vi "BodeMagnitudePlot.vi"() -> ()   [LabVIEW 2014]
uses:
  <vilib>/imath/engines/lvmath2/RunTimeEngine/Managers/WorkSpace/UID Generator.vi
  <vilib>/imath/engines/lvmath2/RunTimeEngine/RunTimeType/NIMS_RunTimeType_From StrictType (excl LVString).vi
  <instcachedir>/0/NIMS_RunTimeType_From StrictType (excl LVString)_15A5391EEA9C4AACB9955AC755B83D29.lvgen/NIMS_RunTimeType_From StrictType (excl LVString)_15A5391EEA9C4AACB9955AC755B83D29_000.vi
  <vilib>/imath/engines/lvmath2/RunTimeEngine/LocalVariableDefStatement/MC_LocalVariableDefStatement_Display.vi
  <vilib>/imath/engines/lvmath2/RunTimeEngine/Managers/SymbolTable/Clear UID.vi
  <vilib>/imath/engines/lvmath2/RunTimeEngine/NodeEndStatement/NIMS_NodeEndStatement_Output.vi
  <instcachedir>/0/NIMS_NodeEndStatement_Output_53EC0D466D134D7ABD903AC30B43404B.lvgen/NIMS_NodeEndStatement_Output_53EC0D466D134D7ABD903AC30B43404B_001.vi
  <vilib>/imath/engines/lvmath2/RunTimeEngine/ErrorHandling/NIMS_Finalize Error.vi
  <vilib>/Analysis/NI_AALPro.lvlib
  <vilib>/imath/engines/lvmath2/RunTimeEngine/Managers/SymbolTable/NIMS_WorkSpace.lvlib
panel:
  out "Outputs":cluster{"freq":dbl[], "G":dbl[]}
  out "XY Graph":cluster{"freq":dbl[], "G":dbl[]}(graph)
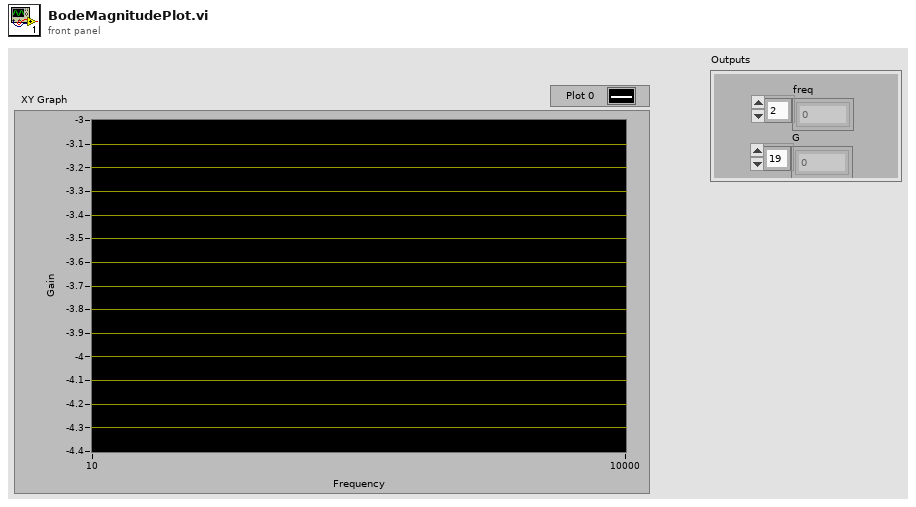
[diagram p1: front panel]
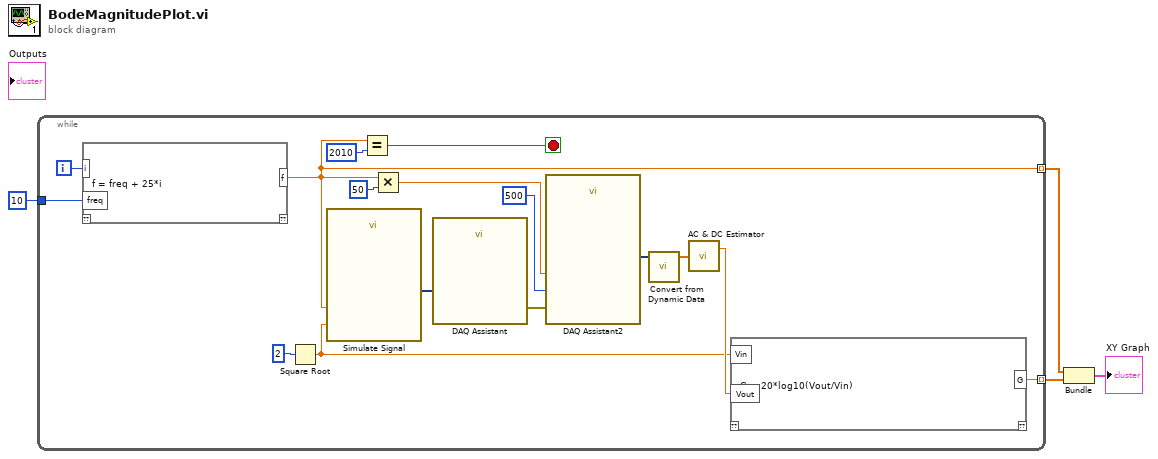
[diagram p0: block diagram]
diagram:
  n1 = while {
    tunnel: 10 -> [w11]
    tunnel: [w10] -> w3 mode=indexing
    tunnel: [w5] -> w1 mode=indexing
    i -> [w12]
    stop <- w8 stop-if-true
    n2 = mathscript code="f = freq + 25*i"("i"=w12, "freq"=w11) -> ("f"=w5:dbl)  [unwired: 1 in, 1 out]
    n3 = Square Root(x=2) -> (sqrt(x)=w6:dbl)
    n4 = call "Simulate Signal"("Frequency"=w5, "Amplitude"=w6) -> ("Sine"=w13:dynamicdata)  [unwired: 12 in, 1 out]
    n5 = Equal?(x=w5, y=2010) -> (x = y?=w8:bool)
    n6 = Multiply(x=w5, y=50) -> (x*y=w17:dbl)
    n7 = call "DAQ Assistant"("data"=w13) -> ("error out"=w16:errorcluster)  [unwired: 16 in, 2 out]
    n8 = call "DAQ Assistant2"("rate"=w17, "number of samples"=500, "error in"=w16) -> ("data"=w15:dynamicdata)  [unwired: 14 in, 2 out]
    n9 = call "Convert from Dynamic Data"("Dynamic Data Type"=w15) -> ("Array"=w14:dbl[])  [unwired: 3 in]
    n10 = call <vilib>:"AC & DC Estimator.vi"("Signal (V)"=w14) -> ("AC estimate (Vrms)"=w7:dbl)  [unwired: 1 out]
    n11 = mathscript code="G = 20*log10(Vout/Vin)"("Vin"=w6, "Vout"=w7) -> ("G"=w10:dbl)  [unwired: 1 in, 1 out]
  }
  n12 = Bundle(w1, w3) -> (→"XY Graph":cluster{dbl[], dbl[]})  [unwired: 1 in]
